vi "Child Inheritance.vi"(8 "error in (no error)":errorcluster, 9 "Child In":refnum<class "System Actor.lvclass">, 11 "Ancestor In":refnum<class "System Actor.lvclass">) -> (0 "error out":errorcluster, 3 "Child Out":refnum<class "System Actor.lvclass">)   [LabVIEW 2019, in "System Actor.lvclass"]
uses:
  System Actor.lvclass
  System Actor.lvclass/System Actor.ctl
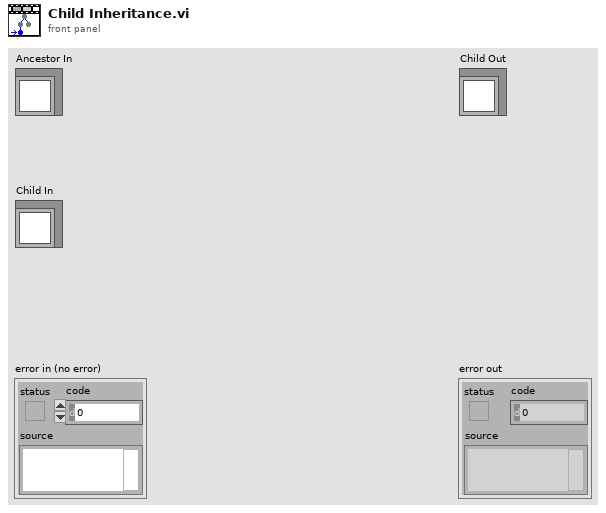
[diagram p1: front panel]
types:
  T1 = typedef "Rendezvous RefNum" = refnum<k1>
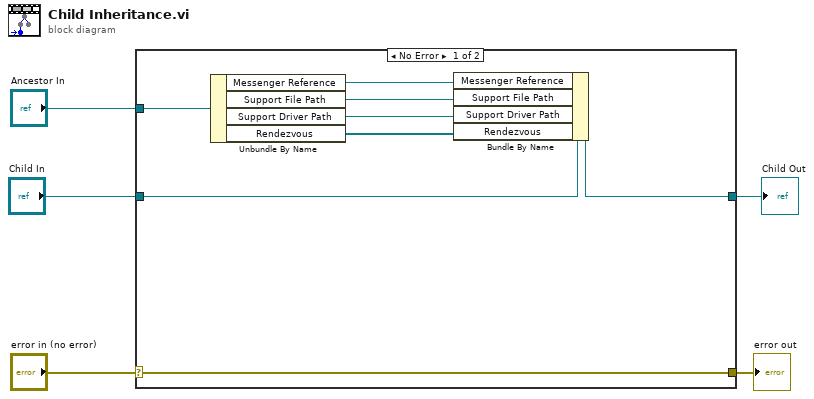
[diagram p0: block diagram]
diagram:
  n1 = case shown="No Error" "error in (no error)" {
    selector: "error in (no error)" -> [w13 w15]
    tunnel: [w13 w15] -> w4
    tunnel: [w10 w14] -> w2
    tunnel: "Ancestor In" -> [w12 _]
    tunnel: "Child In" -> [w11 w14]
    frame No Error {
      n2 = Unbundle By Name(w12) -> ("Messenger Reference"=w9:refnum<data-value>, "Support File Path"=w8:path, "Support Driver Path"=w7:path, "Rendezvous"=w6:T1[])
      n3 = Bundle By Name(cluster=w11, "Messenger Reference"=w9, "Support File Path"=w8, "Support Driver Path"=w7, "Rendezvous"=w6) -> (w10:refnum<class "System Actor.lvclass">)
    }
    frame Error {
    }
  }
  "error out" <- w4
  "Child Out" <- w2
